vi "Create Waveform Cluster.vi"   [LabVIEW 2020]
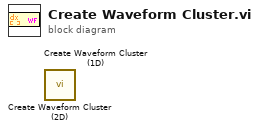
[diagram p0: block diagram]
diagram:
  n1 = call "Create Waveform Cluster (2D).vi"() -> ()  [unwired: 5 in, 1 out]
  n2 = call "Create Waveform Cluster (1D).vi"() -> ()  [unwired: 5 in, 1 out]
